vi "AdvServo example.vi"() -> ()   [LabVIEW 2012]
panel:
  out "error out":errorcluster
  in  "Engaged":bool
  in  "Motor Position":dbl(slide) scale=0.0..200.0
  in  "Which Motor to Control":i32=1 min=1 max=8 step=1
  in  "Stop":bool
  out "Serial Number":i32
  out "Attached":bool
  out "Setups":T1(array[cluster]) {"Motor Position Indicator" scale=0.0..200.0; "Acceleration" format="%#_6f"}
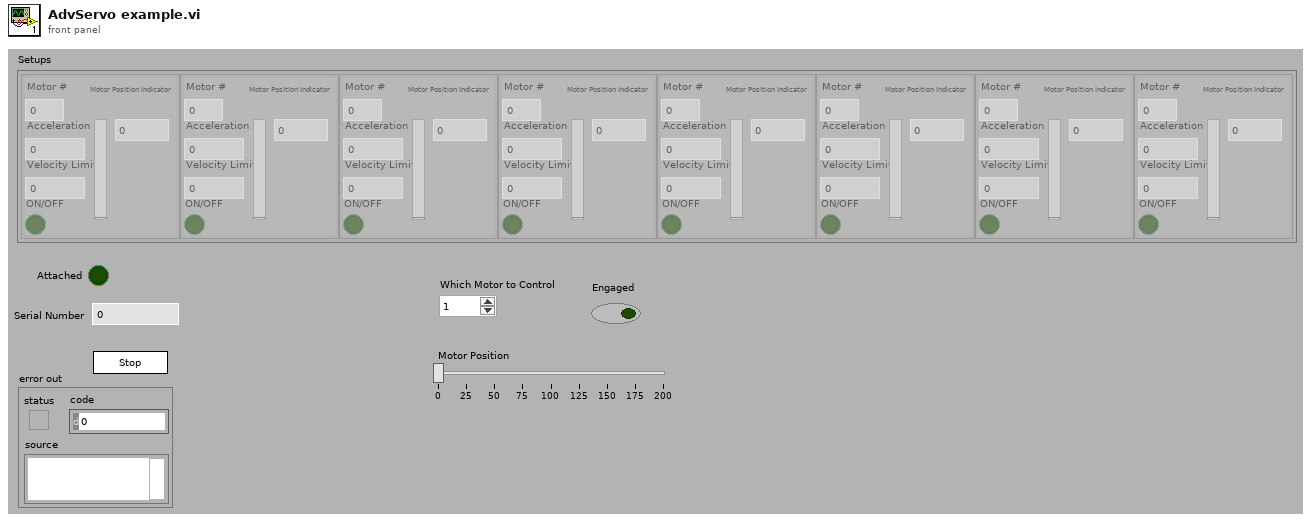
[diagram p1: front panel]
types:
  T1 = cluster{"Motor #":i32, "Acceleration":dbl, "Velocity Limit":dbl, "ON/OFF":bool, "Motor Position Indicator":dbl}[]
  T2 = cluster{i32, "acce_out":dbl, "vellim_out":dbl, "Attached":bool, dbl}
  T3 = cluster{"Motor #":i32, "Acceleration":dbl, "Velocity Limit":dbl, "ON/OFF":bool, "Motor Position Indicator":dbl}
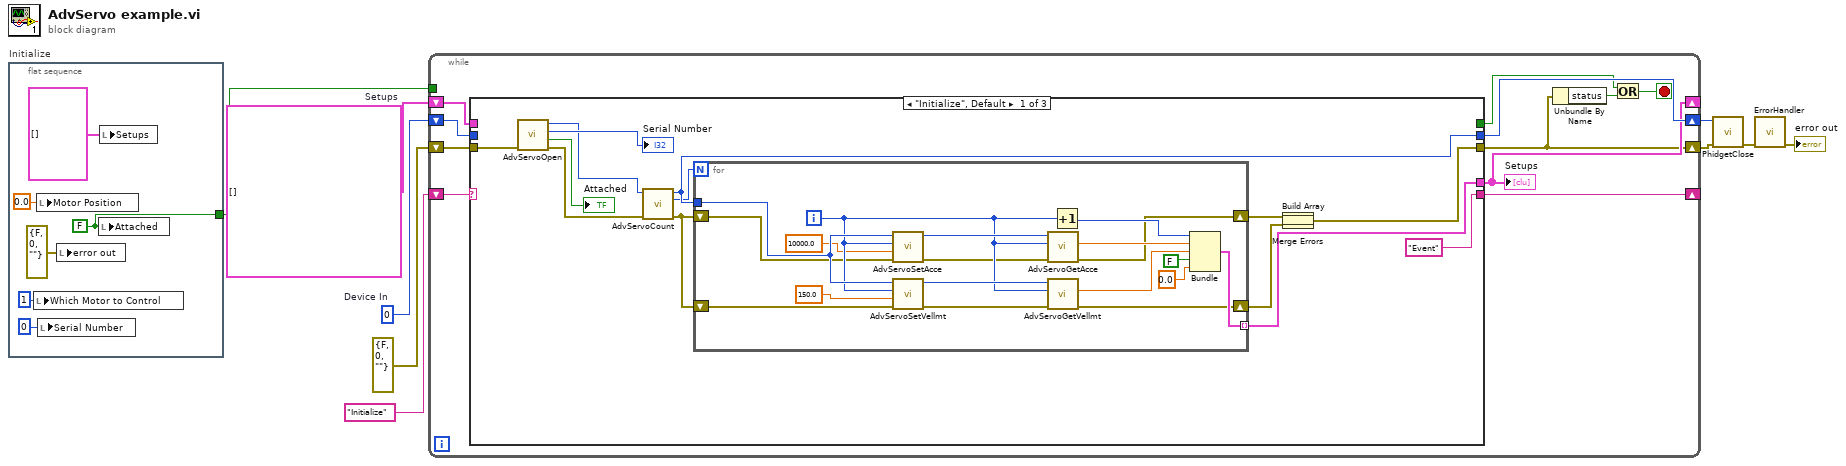
[diagram p0: block diagram]
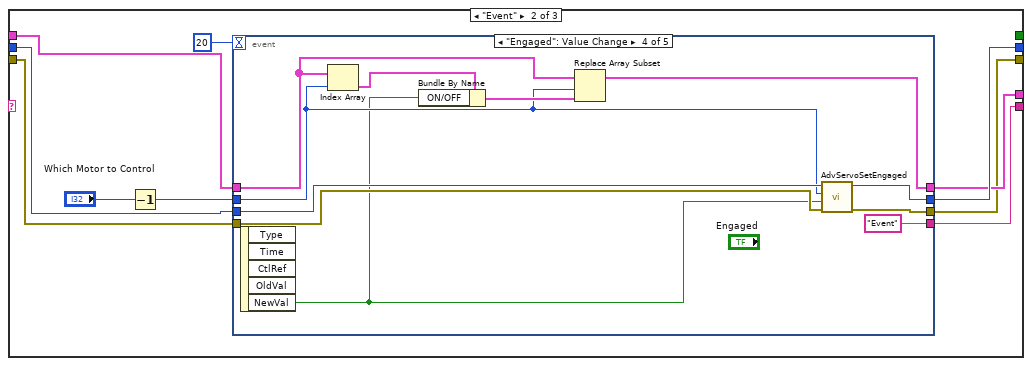
[diagram p2: hidden frame]
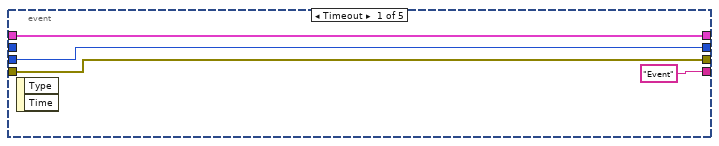
[diagram p3: hidden frame]
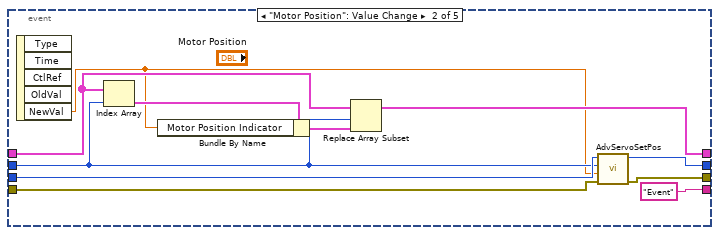
[diagram p4: hidden frame]
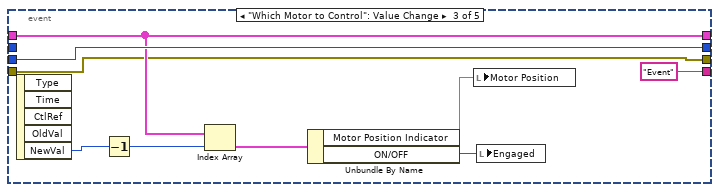
[diagram p5: hidden frame]
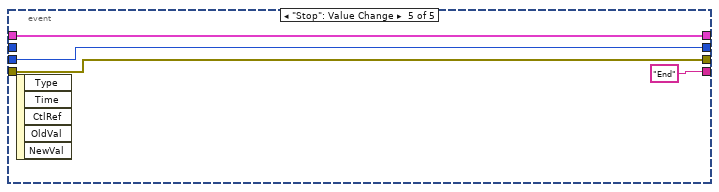
[diagram p6: hidden frame]
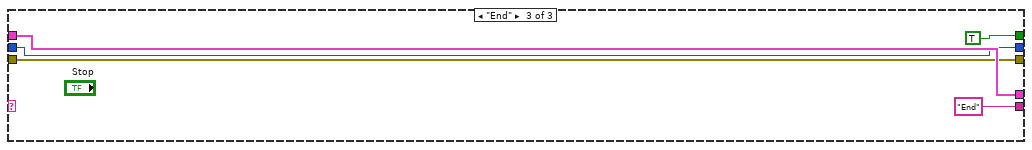
[diagram p7: hidden frame]
diagram:
  w7 = T1 []  # Setups
  w8 = 0  # Device In
  n1 = flat-sequence "Initialize" {
    tunnel: [w10] -> w1
    frame #0 {
      w10 = FALSE ("Attached")
      n2 = local write "Which Motor to Control"(1 ("Which Motor to Control")) -> ()
      n3 = local write "Motor Position"(0.0 ("Motor Position")) -> ()
      n4 = local write "Serial Number"(0 ("Serial Number")) -> ()
      n5 = local write "error out"(errorcluster {"status"=FALSE, "code"=0, "source"=""} ("error out")) -> ()
      n6 = local write "Attached"(w10) -> ()
      n7 = local write "Setups"(T1 [] ("Setups")) -> ()
    }
  }
  n8 = while {
    shift-right: [w23] -> _
    shift-left: "Initialize" -> [w26]
    shift-right: [w25] -> w5
    shift-left: w8 -> [w24]
    shift-right: [w22] -> _
    shift-left: w7 -> [w21]
    shift-right: [w17] -> w4
    shift-left: errorcluster {"status"=FALSE, "code"=0, "source"=""} ("error IO") -> [w20]
    tunnel: w1 -> [_]
    stop <- w19 stop-if-true
    n9 = case shown="\"Initialize\", Default" w26 {
      tunnel: [w37 w66 w109] -> w25
      tunnel: w24 -> [_ w67 w109]
      tunnel: ["Event" w68 "End"] -> w23
      tunnel: [_ _ TRUE] -> w18
      tunnel: [w34 w61 w110] -> w22
      tunnel: w21 -> [_ w62 w110]
      tunnel: w20 -> [w33 w60 w108]
      tunnel: [w28 w59 w108] -> w17
      frame "Initialize", Default {
        n10 = call "AdvServoOpen.vi"("error in"=w33) -> ("error out"=w32:errorcluster, "Attached?"=→"Attached":bool, "Serial Number Return"=→"Serial Number":i32, "Device Out"=w38:i32)  [unwired: 7 in]
        n11 = call "AdvServoCount.vi"("error in (no error)"=w32, "Device In"=w38) -> ("error out"=w31:errorcluster, "count"=w35:i32, "Device Out"=w37:i32)  [unwired: 7 in]
        n12 = for {
          N: w35 -> [_]
          tunnel: w37 -> [w54]
          tunnel: [w57] -> w34 mode=indexing
          shift-right: [w44] -> w29
          shift-left: w31 -> [w46]
          shift-right: [w41] -> w30
          shift-left: w31 -> [w43]
          i -> [w51]
          n13 = call "AdvServoSetAcce.vi"("error in (no error)"=w46, "acce_in"=10000.0, "index"=w51, "Device In"=w54) -> ("error out"=w45:errorcluster, "Device Out"=w55:i32)  [unwired: 5 in]
          n14 = call "AdvServoSetVellmt.vi"("error in (no error)"=w43, "vel_in"=150.0, "index"=w51, "Device In"=w54) -> ("error out"=w42:errorcluster, "Device Out"=w52:i32)  [unwired: 5 in]
          n15 = call "AdvServoGetAcce.vi"("error in (no error)"=w45, "index"=w51, "Device In"=w55) -> ("error out"=w44:errorcluster, "acce_out"=w58:dbl)  [unwired: 5 in, 1 out]
          n16 = call "AdvServoGetVellmt.vi"("error in (no error)"=w42, "index"=w51, "Device In"=w52) -> ("error out"=w41:errorcluster, "vellim_out"=w53:dbl)  [unwired: 5 in, 1 out]
          n17 = Increment(x=w51) -> (x+1=w56:i32)
          n18 = Bundle(w56, "acce_out"=w58, "vellim_out"=w53, "Attached"=FALSE, 0.0) -> (w57:T2)  [unwired: 1 in]
        }
        n19 = Build Array(w29, w30) -> (w27:errorcluster[])
        n20 = Merge Errors(w27) -> (w28:errorcluster)
      }
      frame "Event" {
        n21 = Decrement(x="Which Motor to Control") -> (x-1=w63:i32)
        n22 = event shown="[3] \"Engaged\": Value Change" {
          selector: _ -> [_ _ _ _ _]
          dyn-events: _ -> [_ _ _ _ _]
          timeout: 20 -> [_ _ _ _ _]
          tunnel: ["Event" "Event" "Event" "Event" "End"] -> w68
          tunnel: w67 -> [w71 w83 w90 w103 w106]
          tunnel: [w71 w76 w90 w102 w106] -> w66
          tunnel: w63 -> [_ w77 _ w97 _]
          tunnel: w62 -> [w70 w79 w89 w98 w105]
          tunnel: [w70 w78 w89 w96 w105] -> w61
          tunnel: w60 -> [w69 w74 w84 w95 w104]
          tunnel: [w69 w73 w84 w94 w104] -> w59
          event Timeout {
            n23 = event-data() -> ()  [unwired: 1 in, 2 out]
          }
          event "Motor Position": Value Change {
            n24 = event-data() -> ("NewVal"=w75:dbl)  [unwired: 1 in, 4 out]
            n25 = Index Array(array=w79, index=w77) -> (element=w81:T3)
            n26 = Bundle By Name(cluster=w81, "Motor Position Indicator"=w75) -> (w80:T3)
            n27 = Replace Array Subset(array=w79, new element=w80, index=w77) -> (w78:T1)
            n28 = call "AdvServoSetPos.vi"("error in (no error)"=w74, "pos_in"=w75, "index"=w77, "Device In"=w83) -> ("error out"=w73:errorcluster, "Device Out"=w76:i32)  [unwired: 5 in]
          }
          event "Which Motor to Control": Value Change {
            n29 = event-data() -> ("NewVal"=w88:i32)  [unwired: 1 in, 4 out]
            n30 = Decrement(x=w88) -> (x-1=w87:i32)
            n31 = Index Array(array=w89, index=w87) -> (element=w91:T3)
            n32 = Unbundle By Name(w91) -> ("Motor Position Indicator"=w85:dbl, "ON/OFF"=w86:bool)
            n33 = local write "Motor Position"(w85) -> ()
            n34 = local write "Engaged"(w86) -> ()
          }
          event "Engaged": Value Change {
            n35 = event-data() -> ("NewVal"=w93:bool)  [unwired: 1 in, 4 out]
            n36 = Index Array(array=w98, index=w97) -> (element=w100:T3)
            n37 = Bundle By Name(cluster=w100, "ON/OFF"=w93) -> (w99:T3)
            n38 = Replace Array Subset(array=w98, new element=w99, index=w97) -> (w96:T1)
            n39 = call "AdvServoSetEngaged.vi"("error in (no error)"=w95, "SetEngaged"=w93, "index"=w97, "Device In"=w103) -> ("error out"=w94:errorcluster, "Device Out"=w102:i32)  [unwired: 5 in]
          }
          event "Stop": Value Change {
            n40 = event-data() -> ()  [unwired: 1 in, 5 out]
          }
        }
      }
      frame "End" {
      }
    }
    "Setups" <- w22
    n41 = Unbundle By Name(w17) -> ("status"=w16:bool)
    n42 = Or(x=w18, y=w16) -> (x .or. y?=w19:bool)
  }
  n43 = call "PhidgetClose.vi"("error in"=w4, "Device In"=w5) -> ("error out"=w3:errorcluster)  [unwired: 9 in]
  n44 = call "ErrorHandler.vi"("error in"=w3) -> ("error out"=→"error out":errorcluster)  [unwired: 9 in, 1 out]
